vi "FlatUIWindow.vi"() -> ()   [LabVIEW 2019]
uses:
  user32.dll
panel:
  in  "stop":bool
  out "Flat UI Window Title":bool
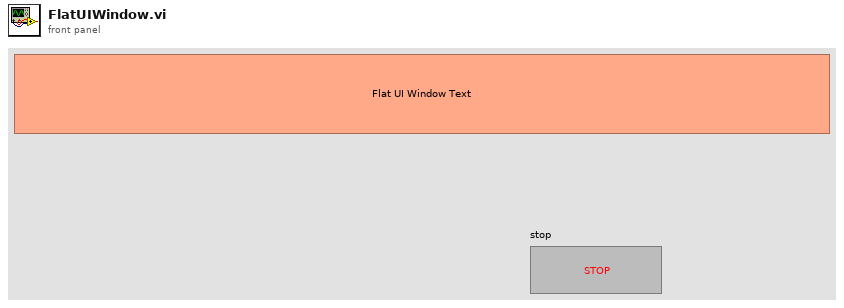
[diagram p1: front panel]
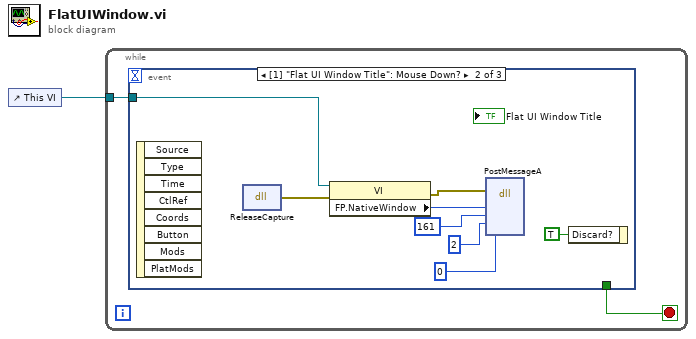
[diagram p0: block diagram]
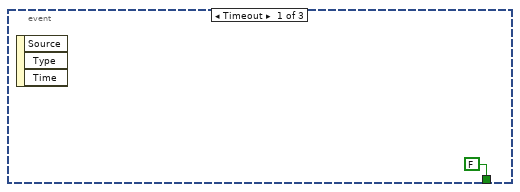
[diagram p2: hidden frame]
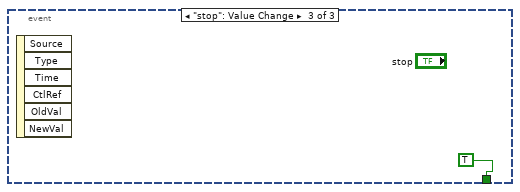
[diagram p3: hidden frame]
diagram:
  n1 = control-ref of="This VI"() -> (w1:refnum<vi>)
  n2 = while {
    tunnel: w1 -> [w3]
    stop <- w2 stop-if-true
    n3 = event shown="[1] \"Flat UI Window Title\": Mouse Down?" {
      selector: _ -> [_ _ _]
      dyn-events: _ -> [_ _ _]
      timeout: _ -> [_ _ _]
      tunnel: w3 -> [_ w12 _]
      tunnel: [FALSE _ TRUE] -> w2
      event Timeout {
        n4 = event-data() -> ()  [unwired: 1 in, 3 out]
      }
      event "Flat UI Window Title": Mouse Down? {
        n5 = event-data() -> ()  [unwired: 1 in, 8 out]
        n6 = dll-call lib="user32.dll" fn="ReleaseCapture"() -> (error out=w10:errorcluster)  [unwired: 4 in, 1 out]
        n7 = property class="VI"(reference=w12, error in=w10) -> (error out=w5:errorcluster, "FP.NativeWindow"=w9:u64)  [unwired: 1 out]
        n8 = dll-call lib="user32.dll" fn="PostMessageA"(error in=w5, "arg1"=w9, "arg2"=161, "arg3"=2 ("arg2"), "arg4"=0 ("arg2")) -> ()  [unwired: 7 in, 2 out]
        n9 = event-data("Discard?"=TRUE) -> ()  [unwired: 1 in, 1 out]
      }
      event "stop": Value Change {
        n10 = event-data() -> ()  [unwired: 1 in, 6 out]
      }
    }
  }
